vi "太阳能控制器界面.vi"() -> ()   [LabVIEW 2016, in "环境动力监测库.lvlib"]
uses:
  <vilib>/Utility/miscctls.llb/LVPointTypeDef.ctl
  <vilib>/Utility/config.llb/NI_LVConfig.lvlib
  <vilib>/ptbypt/NI_PtbyPt.lvlib
panel:
  out "串口":string
  in  "串口启用 2":bool caption="串口启用"
  in  "串口启用":bool
  in  "报警设置":bool
  in  "MPPT-24 串口":refnum<visa-resource-name> caption="MPPT-24"
  in  "MPPT-12 串口":refnum<visa-resource-name> caption="MPPT-12"
  out "充放电信息 2":T1 caption="充放电信息_KWH" {"总累计充电量" format="%.2f"; "当年累计充电量" format="%.2f"; "当月累计充电量" format="%.2f"; "当日累计充电量" format="%.2f"; "当年累计用电量" format="%.2f"; "当月累计用电量" format="%.2f"; "当日累计用电量" format="%.2f"}
  out "状态 2":string caption="状态"
  out "状态":string
  out "充放电信息":T1 caption="充放电信息_KWH" {"总累计充电量" format="%.2f"; "当年累计充电量" format="%.2f"; "当月累计充电量" format="%.2f"; "当日累计充电量" format="%.2f"; "当年累计用电量" format="%.2f"; "当月累计用电量" format="%.2f"; "当日累计用电量" format="%.2f"}
  out "通讯状态 3":bool
  out "通讯状态 2":bool
  out "控制器信息 2":cluster{"设备温度℃":dbl} caption="控制器信息"
  out "直流负载信息 2":cluster{"负载电压V":dbl, "负载电流A":dbl, "负载功率W":dbl} caption="直流负载信息"
  out "蓄电池信息 2":T2 caption="蓄电池信息"
  out "阵列信息 2":cluster{"阵列电压V":dbl, "阵列电流A":dbl, "发电功率W":dbl} caption="阵列信息"
  out "控制器信息":cluster{"设备温度℃":dbl}
  out "直流负载信息":cluster{"负载电压V":dbl, "负载电流A":dbl, "负载功率W":dbl}
  out "蓄电池信息":T2
  out "阵列信息":cluster{"阵列电压V":dbl, "阵列电流A":dbl, "发电功率W":dbl}
  # "MPPT-12"
  # "MPPT-24"
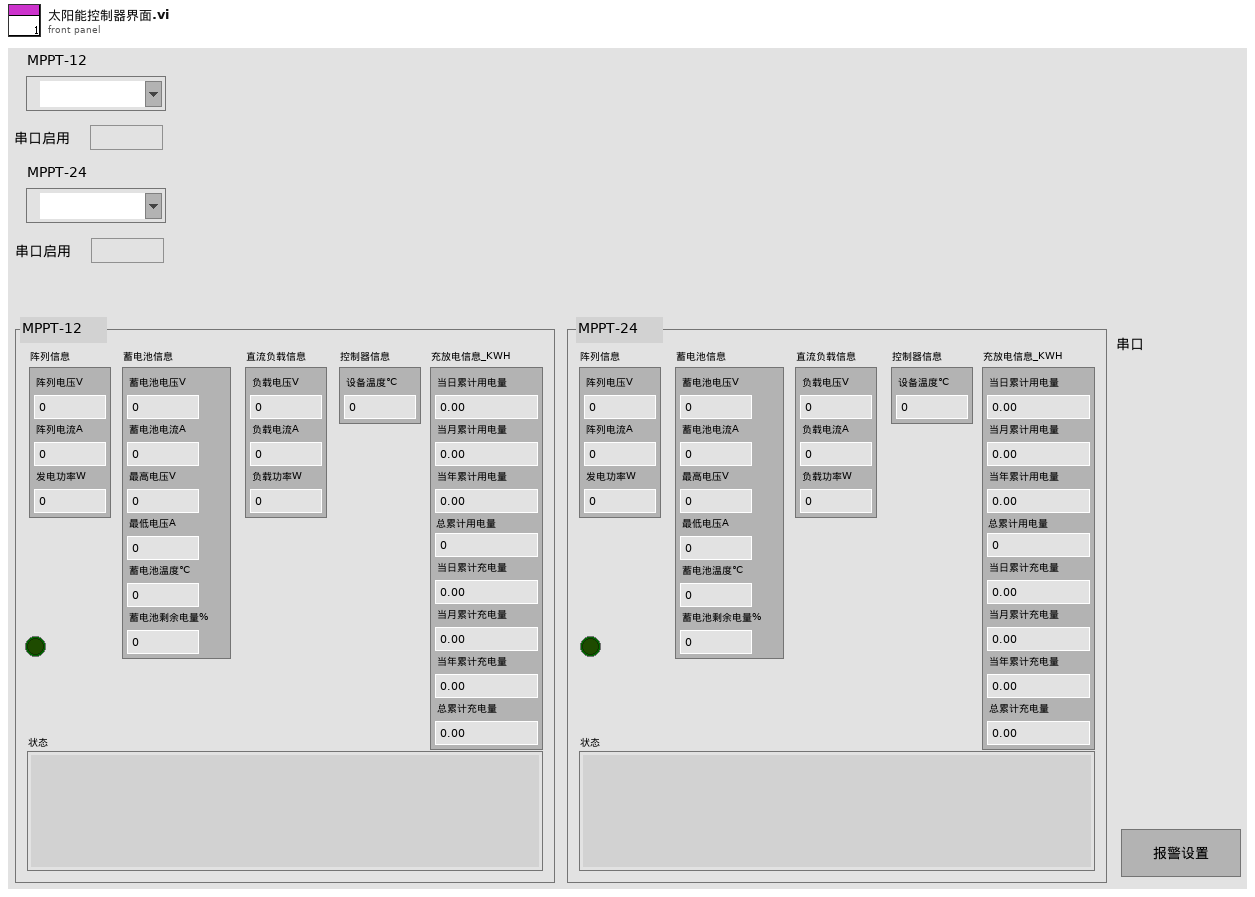
[diagram p1: front panel]
types:
  T1 = cluster{"当日累计用电量":sgl, "当月累计用电量":sgl, "当年累计用电量":sgl, "总累计用电量":sgl, "当日累计充电量":sgl, "当月累计充电量":sgl, "当年累计充电量":sgl, "总累计充电量":sgl}
  T2 = cluster{"蓄电池电压V":dbl, "蓄电池电流A":dbl, "最高电压V":dbl, "最低电压A":dbl, "蓄电池温度℃":dbl, "蓄电池剩余电量%":dbl}
  T3 = cluster{"监测项描述:输出":string, "连接方式":enum16{"串口", "TCP"}, "端口":string, "IP address:":string, "Port:":string, "站号":u64, "传感器型号":string, "波特率":u64, "data bits":u64, "停止位":u16, "奇偶校验":u16}
  T4 = typedef "LVPointTypeDef.ctl" = cluster{"Horizontal":i16, "Vertical":i16}
  T5 = typedef "NI_LVConfig.lvlib/Config Data RefNum.ctl" = refnum<k1>
  T6 = cluster{"时间":timestamp, "阵列电压_V":dbl, "阵列电流_A":dbl, "发电功率_W":dbl, "蓄电池电压_V":dbl, "蓄电池电流_A":dbl, "最高电压_V":dbl, "最低电压_A":dbl, "蓄电池温度_℃":dbl, "蓄电池剩余电量_%":dbl, "负载电压_V":dbl, "负载电流_A":dbl, "负载功率_W":dbl, "设备温度_℃":dbl, "当日累计用电量_KWH":dbl, "当月累计用电量_KWH":dbl, "当年累计用电量_KWH":dbl, "总累计用电量_KWH":dbl, "当日累计充电量_KWH":dbl, "当月累计充电量_KWH":dbl, "当年累计充电量_KWH":dbl, "总累计充电量_KWH":dbl}
  T7 = typedef "LVDateTimeRec.ctl" = cluster{"秒数的小数部分":dbl, "秒":i32, "分":i32, "时":i32, "日":i32, "月":i32, "年":i32, "天数（周）":i32, "天数（年）":i32, "DST":i32}
  T8 = cluster{"漏水监测输出":bool, "门禁监测输出":bool, "温湿度监测输出":bool, "烟雾监测输出":bool, "空调监测输出":bool, "自动重合闸输出":bool, "红外入侵输出":bool, "振动输出":bool, "UPS输出":bool, "蓄电池输出":bool, "定位输出":bool}
  T9 = cluster{"状态":cluster{"蓄电池状态":string, "阵列状态":string, "充电状态":string, "负载状态":string, "设备状态":string}, "充放电信息":cluster{"当日累计用电量":sgl, "当月累计用电量":sgl, "当年累计用电量":sgl, "总累计用电量":sgl, "当日累计充电量":sgl, "当月累计充电量":sgl, "当年累计充电量":sgl, "总累计充电量":sgl}, "控制器信息":cluster{"设备温度℃":dbl}, "蓄电池信息":cluster{"蓄电池电压V":dbl, "蓄电池电流A":dbl, "最高电压V":dbl, "最低电压A":dbl, "蓄电池温度℃":dbl, "蓄电池剩余电量%":dbl}, "阵列信息":cluster{"阵列电压V":dbl, "阵列电流A":dbl, "发电功率W":dbl}, "直流负载信息":cluster{"负载电压V":dbl, "负载电流A":dbl, "负载功率W":dbl}, "error out":errorcluster}
  T10 = cluster{"市电":cluster{"电压:":u16, "电流：":dbl, "状态":bool}, "UPS":cluster{"输入电压:":sgl, "输出电压:":sgl, "电池电量:":u8, "电量":u16, "状态":bool}, "蓄电池":cluster{"电压:":sgl, "电流:":sgl, "电池电量:":u8, "电量":u16, "状态":bool}}
  T11 = enum8{"Enabled", "Disabled", "Disabled and Grayed Out"}
  T12 = cluster{"蓄电池状态":string, "阵列状态":string, "充电状态":string, "负载状态":string, "设备状态":string}
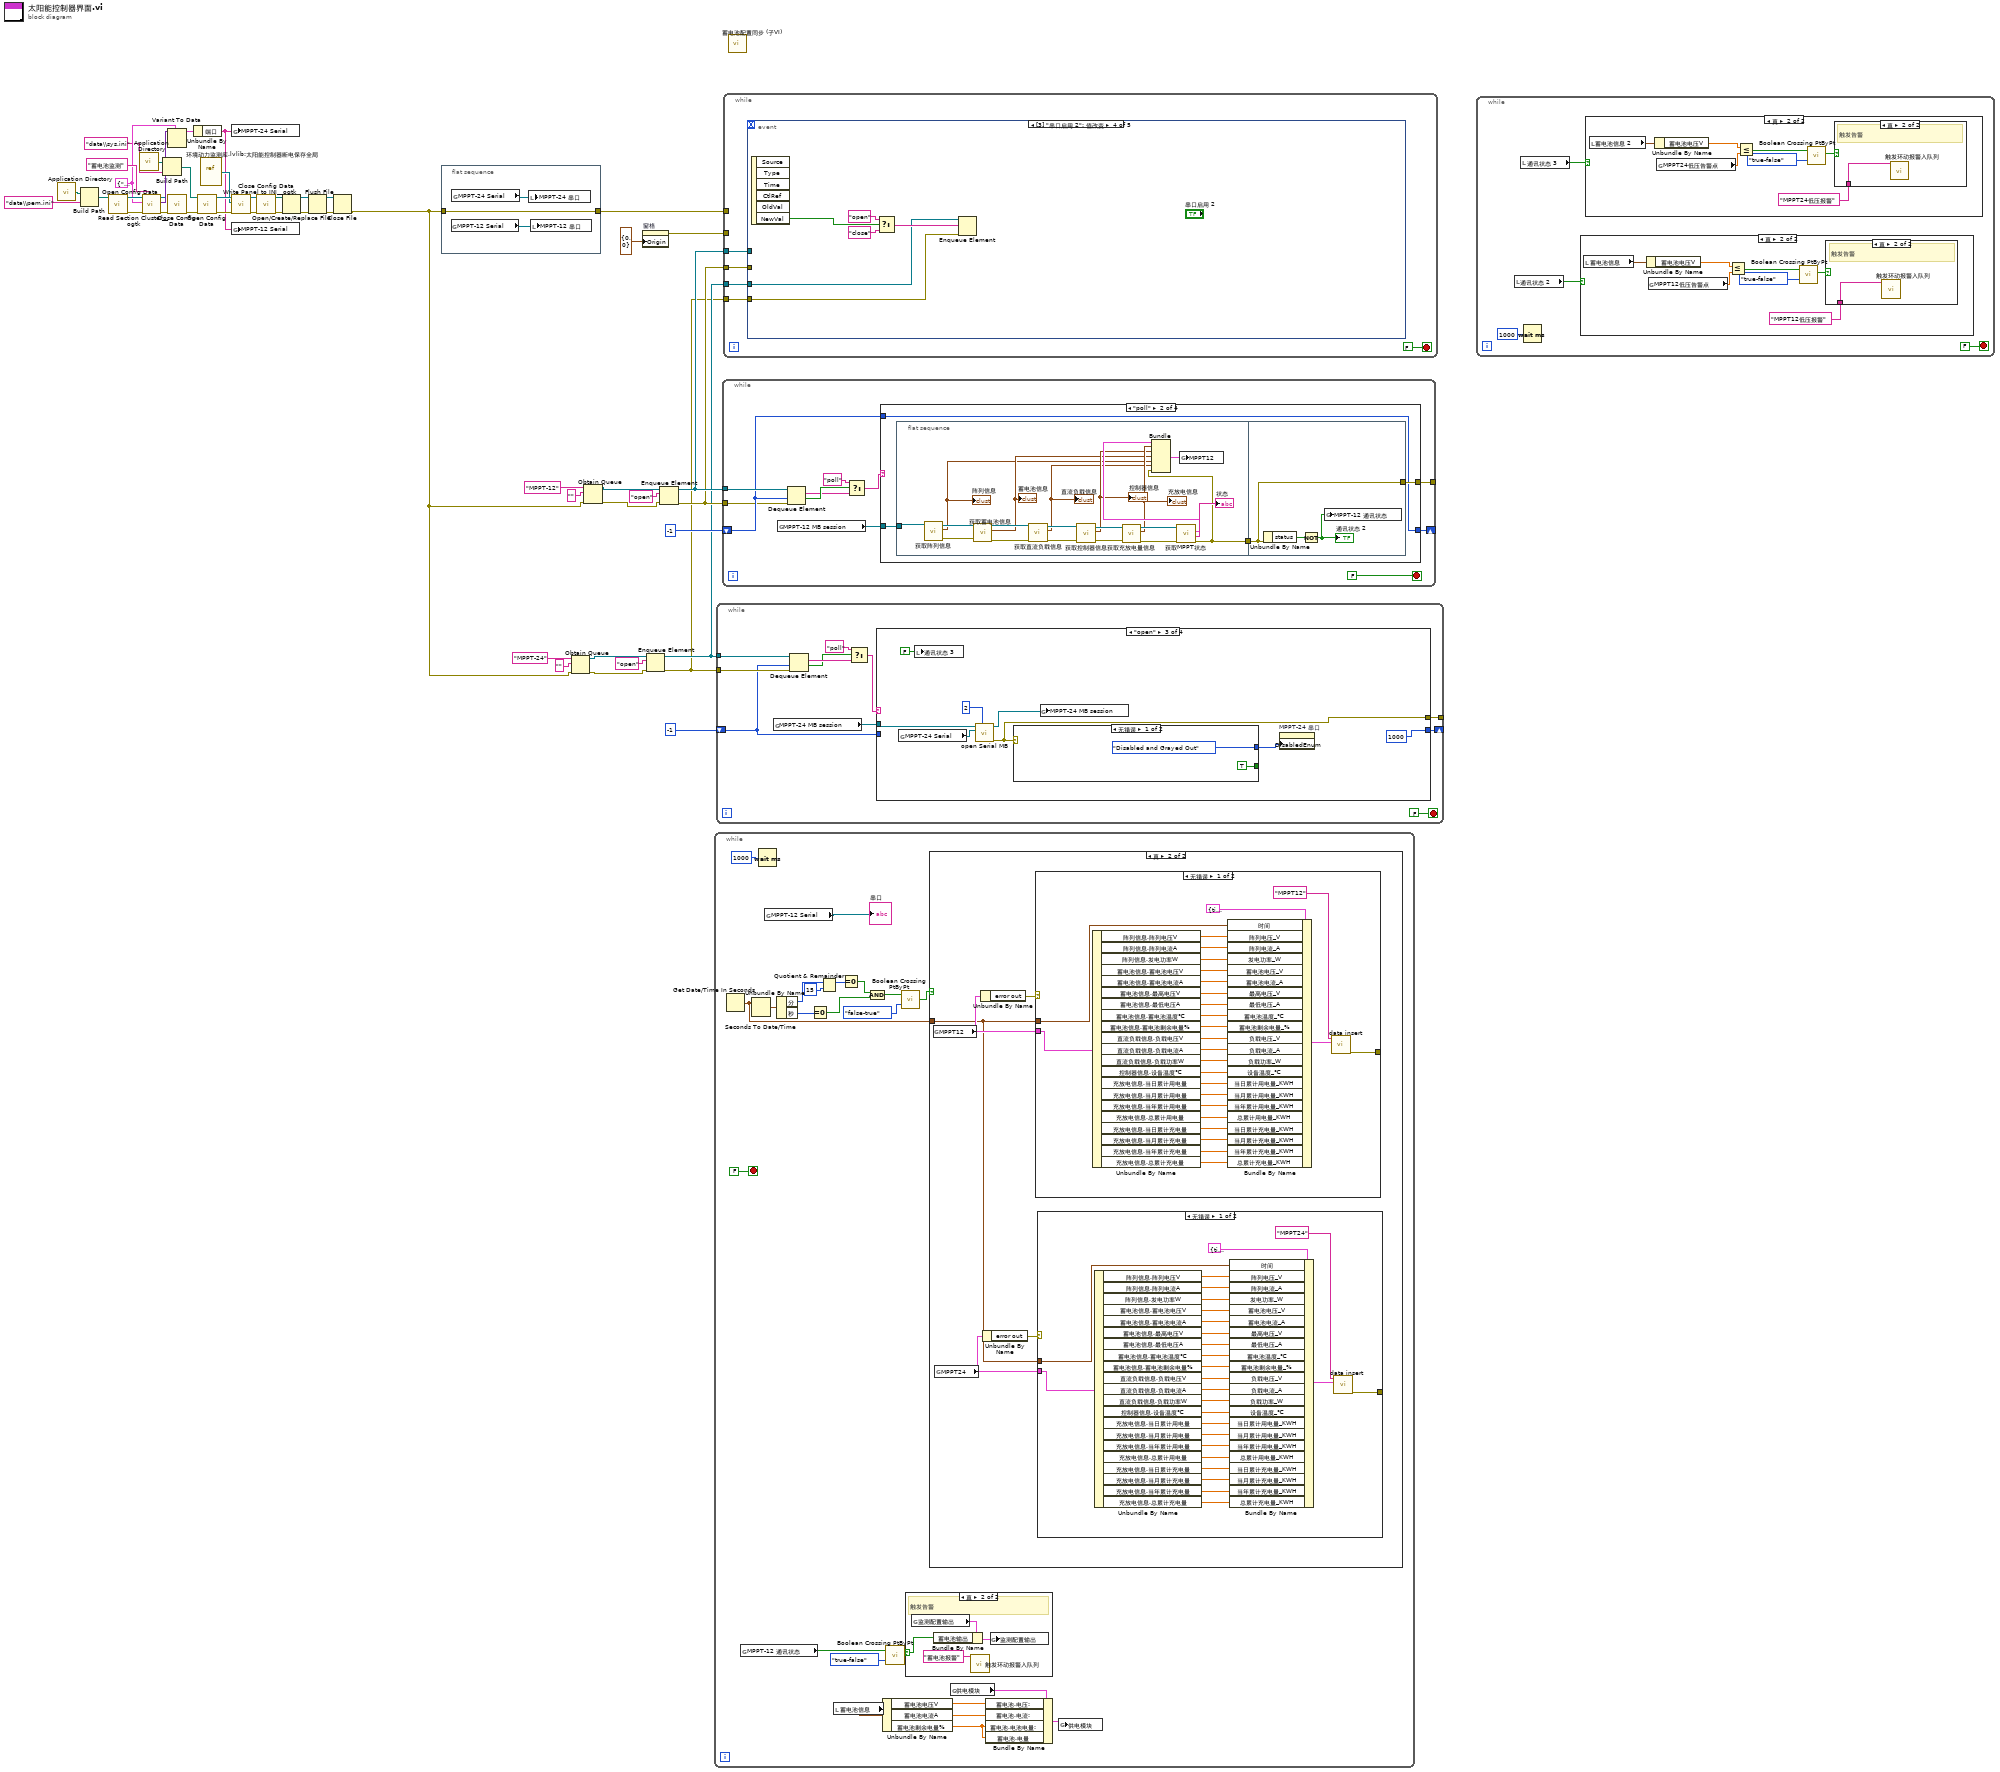
[diagram p0: block diagram]
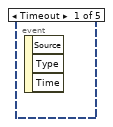
[diagram p10: hidden frame]
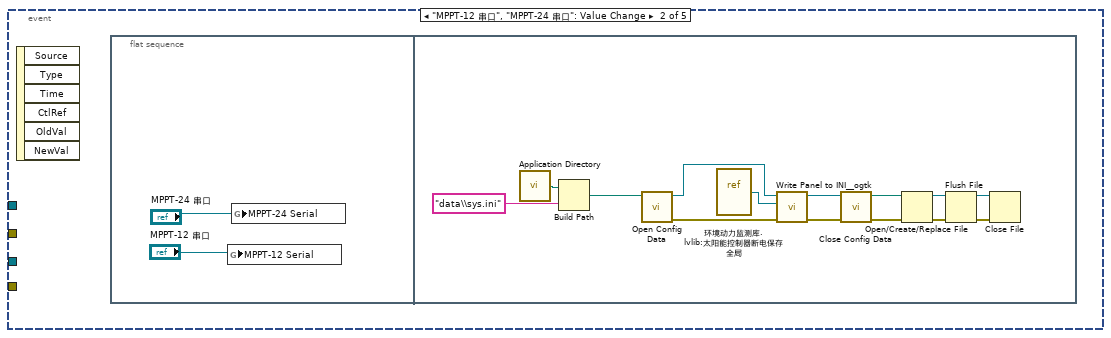
[diagram p11: hidden frame]
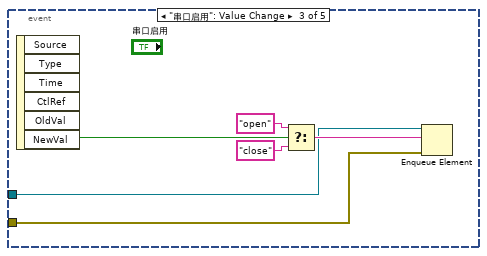
[diagram p12: hidden frame]
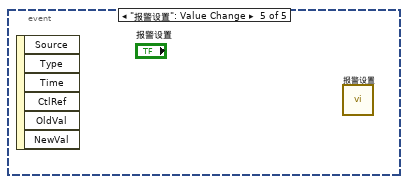
[diagram p13: hidden frame]
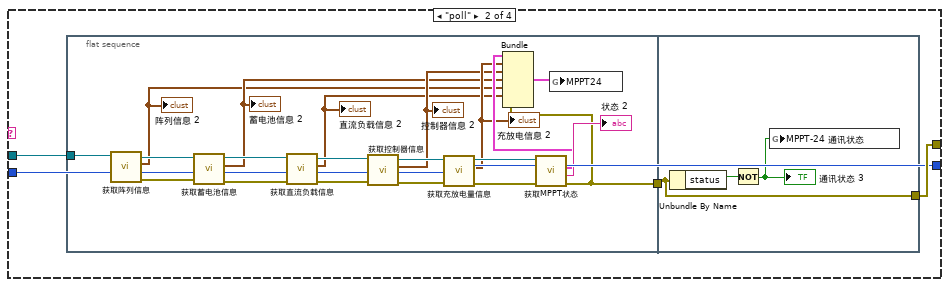
[diagram p15: hidden frame]
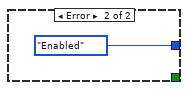
[diagram p16: hidden frame]
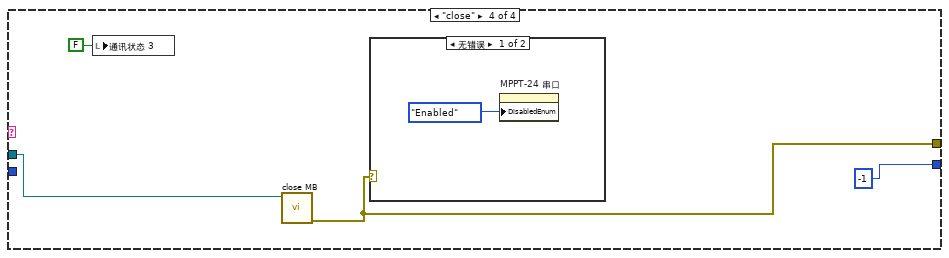
[diagram p17: hidden frame]
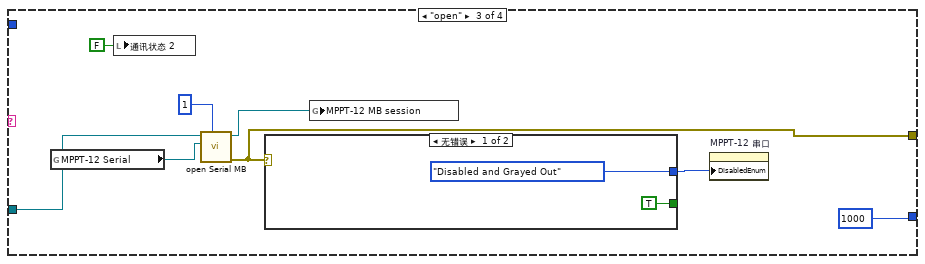
[diagram p20: hidden frame]
diagram:
  w18 = T3 {"监测项描述:输出"="", "连接方式"=enum."串口", "端口"="", "IP address:"="", "Port:"="", "站号"=19200, "传感器型号"="", "波特率"=19200, "data bits"=8, "停止位"=10, "奇偶校验"=0} ("输入簇")
  n1 = call <vilib>:"Application Directory.vi"() -> ("Application Directory"=w22:path)
  n2 = Build Path(base path=w22, name or relative path="data\\pem.ini" ("名称或相对路径")) -> (appended path=w21:path)
  n3 = call <vilib>:"Open Config Data.vi"("configuration file path"=w21) -> ("error out"=w20:errorcluster, "refnum"=w19:T5)  [unwired: 8 in, 1 out]
  n4 = call <vilib>:"Application Directory.vi"() -> ("Application Directory"=w16:path)
  n5 = call <userlib>:"Read Section Cluster__ogtk.vi"("section (optional)"="蓄电池监测", "error in (no error)"=w20, "Section Formatted Cluster Type"=w18, "refnum"=w19) -> ("error out"=w26:errorcluster, "Section Formatted Cluster"=w27:variant, "dup refnum"=w25:T5)  [unwired: 3 in, 2 out]
  n6 = Build Path(base path=w16, name or relative path="data\\sys.ini" ("名称或相对路径")) -> (appended path=w15:path)
  n7 = Variant To Data(type=w18, Variant=w27) -> (data=w28:T3)  [unwired: 1 in, 1 out]
  n8 = call <vilib>:"Close Config Data.vi"("error in (no error)"=w26, "refnum"=w25) -> ("error out"=w4:errorcluster)  [unwired: 8 in, 1 out]
  n9 = Unbundle By Name(w28) -> ("端口"=w2:string)
  n10 = call <vilib>:"Open Config Data.vi"("error in (no error)"=w4, "configuration file path"=w15) -> ("error out"=w12:errorcluster, "refnum"=w14:T5)  [unwired: 7 in, 1 out]
  n11 = vi-ref "环境动力监测库.lvlib:太阳能控制器断电保存全局.vi"() -> (w3:refnum<vi>)
  n12 = global write "太阳能控制器断电保存全局.vi" "MPPT-24 Serial"(w2) -> ()
  n13 = call <userlib>:"Write Panel to INI__ogtk.vi"("error in (no error)"=w12, "VI ref"=w3, "refnum"=w14) -> ("error out"=w11:errorcluster, "refnum out"=w13:T5)  [unwired: 7 in]
  n14 = global write "太阳能控制器断电保存全局.vi" "MPPT-12 Serial"(w2) -> ()
  n15 = call <vilib>:"Close Config Data.vi"("error in (no error)"=w11, "refnum"=w13) -> ("error out"=w6:errorcluster, "file path"=w5:path)  [unwired: 8 in]
  n16 = Open/Create/Replace File(file path (use dialog)=w5, error in=w6) -> (refnum out=w9:refnum<file>, error out=w10:errorcluster)  [unwired: 4 in, 1 out]
  n17 = Flush File(refnum=w9, error in=w10) -> (refnum out=w8:refnum<file>, error out=w7:errorcluster)
  n18 = Close File(refnum=w8, error in=w7) -> (error out=w1:errorcluster)  [unwired: 1 out]
  n19 = flat-sequence {
    tunnel: w1 -> [w48]
    tunnel: [w48] -> w33
    frame #0 {
      n20 = global read "太阳能控制器断电保存全局.vi" "MPPT-12 Serial"() -> (w50:refnum<visa-resource-name>)
      n21 = global read "太阳能控制器断电保存全局.vi" "MPPT-24 Serial"() -> (w49:refnum<visa-resource-name>)
      n22 = local write "MPPT-24 串口"(w49) -> ()
      n23 = local write "MPPT-12 串口"(w50) -> ()
    }
  }
  n24 = Obtain Queue(name (unnamed)="MPPT-24" ("名称（未命名）"), element data type="", error in (no error)=w1) -> (queue out=w35:refnum<queue>, error out=w34:errorcluster)  [unwired: 2 in, 1 out]
  n25 = Obtain Queue(name (unnamed)="MPPT-12" ("名称（未命名）"), element data type="", error in (no error)=w1) -> (queue out=w37:refnum<queue>, error out=w36:errorcluster)  [unwired: 2 in, 1 out]
  n26 = property on="窗格" class="Pane"("Origin"=T4 {"Horizontal"=0, "Vertical"=0} ("原点")) -> (error out=w44:errorcluster)  [unwired: 2 in, 1 out]
  n27 = Enqueue Element(queue=w35, element="open" ("元素"), error in (no error)=w34) -> (queue out=w30:refnum<queue>, error out=w29:errorcluster)  [unwired: 1 in, 1 out]
  n28 = Enqueue Element(queue=w37, element="open" ("元素"), error in (no error)=w36) -> (queue out=w32:refnum<queue>, error out=w31:errorcluster)  [unwired: 1 in, 1 out]
  n29 = while {
    stop <- FALSE stop-if-true
    n30 = Get Date/Time In Seconds() -> (seconds since 1Jan1904=w61:timestamp)
    n31 = global read "太阳能控制器全局.vi" "MPPT-12 通讯状态"() -> (w51:bool)
    n32 = Seconds To Date/Time(time stamp (now)=w61) -> (date time rec=w71:T7)  [unwired: 1 in]
    n33 = Wait (ms)(milliseconds to wait=u32 1000 ("等待时间（毫秒）")) -> ()  [unwired: 1 out]
    n34 = global read "太阳能控制器断电保存全局.vi" "MPPT-12 Serial"() -> (→"串口":refnum<visa-resource-name>)
    n35 = Unbundle By Name(w71) -> ("分"=w70:i32, "秒"=w67:i32)
    n36 = Equal To 0?(x=w67) -> (x = 0?=w65:bool)
    n37 = Quotient & Remainder(x=w70, y=15) -> (x-y*floor(x/y)=w68:i32)  [unwired: 1 out]
    n38 = local read "蓄电池信息"() -> (w55:T2)
    n39 = Equal To 0?(x=w68) -> (x = 0?=w66:bool)
    n40 = And(x=w66, y=w65) -> (x .and. y?=w64:bool)
    n41 = Unbundle By Name(w55) -> ("蓄电池电压V"=w54:dbl, "蓄电池电流A"=w53:dbl, "蓄电池剩余电量%"=w52:dbl)
    n42 = call <vilib>:"Boolean Crossing PtByPt.vi"("direction"=enum16{"either", "false-true", "true-false"}."true-false", "input"=w51) -> ("crossing"=w58:bool)  [unwired: 1 in]
    n43 = call <vilib>:"Boolean Crossing PtByPt.vi"("direction"=enum16{"either", "false-true", "true-false"}."false-true", "input"=w64) -> ("crossing"=w62:bool)  [unwired: 1 in]
    n44 = case shown="真" w58 {
      selector: w58 -> [_ w74]
      frame False {
      }
      frame True {
        # "触发告警"
        n45 = global read "断电保存全局变量.vi" "监测配置输出"() -> (w76:T8)
        n46 = Bundle By Name(cluster=w76, "蓄电池输出"=w74) -> (w75:T8)
        n47 = call "触发环动报警入队列.vi"("报警内容"="蓄电池报警") -> ()  [unwired: 11 in]
        n48 = global write "断电保存全局变量.vi" "监测配置输出"(w75) -> ()
      }
    }
    n49 = case shown="真" w62 {
      tunnel: w61 -> [_ w78]
      frame False {
      }
      frame True {
        n50 = global read "太阳能控制器全局.vi" "MPPT12"() -> (w81:T9)
        n51 = global read "太阳能控制器全局.vi" "MPPT24"() -> (w80:T9)
        n52 = Unbundle By Name(w81) -> ("error out"=w82:errorcluster)
        n53 = Unbundle By Name(w80) -> ("error out"=w79:errorcluster)
        n54 = case shown="无错误" w82 {
          tunnel: w81 -> [w114 _]
          tunnel: w78 -> [w113 _]
          tunnel: [w110 _] -> _
          frame No Error {
            n55 = Unbundle By Name(w114) -> ("阵列信息.阵列电压V"=w116:dbl, "阵列信息.阵列电流A"=w117:dbl, "阵列信息.发电功率W"=w118:dbl, "蓄电池信息.蓄电池电压V"=w119:dbl, "蓄电池信息.蓄电池电流A"=w120:dbl, "蓄电池信息.最高电压V"=w121:dbl, "蓄电池信息.最低电压A"=w122:dbl, "蓄电池信息.蓄电池温度℃"=w123:dbl, "蓄电池信息.蓄电池剩余电量%"=w124:dbl, "直流负载信息.负载电压V"=w125:dbl, "直流负载信息.负载电流A"=w126:dbl, "直流负载信息.负载功率W"=w127:dbl, "控制器信息.设备温度℃"=w128:dbl, "充放电信息.当日累计用电量"=w129:sgl, "充放电信息.当月累计用电量"=w130:sgl, "充放电信息.当年累计用电量"=w131:sgl, "充放电信息.总累计用电量"=w132:sgl, "充放电信息.当日累计充电量"=w133:sgl, "充放电信息.当月累计充电量"=w134:sgl, "充放电信息.当年累计充电量"=w135:sgl, "充放电信息.总累计充电量"=w136:sgl)
            n56 = Bundle By Name(cluster=T6 {"时间"=timestamp(0 s since 1904-01-01), "阵列电压_V"=0.0, "阵列电流_A"=0.0, "发电功率_W"=0.0, "蓄电池电压_V"=0.0, "蓄电池电流_A"=0.0, "最高电压_V"=0.0, "最低电压_A"=0.0, "蓄电池温度_℃"=0.0, "蓄电池剩余电量_%"=0.0, "负载电压_V"=0.0, "负载电流_A"=0.0, "负载功率_W"=0.0, "设备温度_℃"=0.0, "当日累计用电量_KWH"=0.0, "当月累计用电量_KWH"=0.0, "当年累计用电量_KWH"=0.0, "总累计用电量_KWH"=0.0, "当日累计充电量_KWH"=0.0, "当月累计充电量_KWH"=0.0, "当年累计充电量_KWH"=0.0, "总累计充电量_KWH"=0.0} ("data in"), "时间"=w113, "阵列电压_V"=w116, "阵列电流_A"=w117, "发电功率_W"=w118, "蓄电池电压_V"=w119, "蓄电池电流_A"=w120, "最高电压_V"=w121, "最低电压_A"=w122, "蓄电池温度_℃"=w123, "蓄电池剩余电量_%"=w124, "负载电压_V"=w125, "负载电流_A"=w126, "负载功率_W"=w127, "设备温度_℃"=w128, "当日累计用电量_KWH"=w129, "当月累计用电量_KWH"=w130, "当年累计用电量_KWH"=w131, "总累计用电量_KWH"=w132, "当日累计充电量_KWH"=w133, "当月累计充电量_KWH"=w134, "当年累计充电量_KWH"=w135, "总累计充电量_KWH"=w136) -> (w112:T6)
            n57 = call "data insert.vi"("data in"=w112, "table"="MPPT12") -> ("error out"=w110:errorcluster)  [unwired: 9 in]
          }
          frame Error {
          }
        }
        n58 = case shown="无错误" w79 {
          tunnel: w80 -> [w87 _]
          tunnel: w78 -> [w86 _]
          tunnel: [w83 _] -> _
          frame No Error {
            n59 = Unbundle By Name(w87) -> ("阵列信息.阵列电压V"=w89:dbl, "阵列信息.阵列电流A"=w90:dbl, "阵列信息.发电功率W"=w91:dbl, "蓄电池信息.蓄电池电压V"=w92:dbl, "蓄电池信息.蓄电池电流A"=w93:dbl, "蓄电池信息.最高电压V"=w94:dbl, "蓄电池信息.最低电压A"=w95:dbl, "蓄电池信息.蓄电池温度℃"=w96:dbl, "蓄电池信息.蓄电池剩余电量%"=w97:dbl, "直流负载信息.负载电压V"=w98:dbl, "直流负载信息.负载电流A"=w99:dbl, "直流负载信息.负载功率W"=w100:dbl, "控制器信息.设备温度℃"=w101:dbl, "充放电信息.当日累计用电量"=w102:sgl, "充放电信息.当月累计用电量"=w103:sgl, "充放电信息.当年累计用电量"=w104:sgl, "充放电信息.总累计用电量"=w105:sgl, "充放电信息.当日累计充电量"=w106:sgl, "充放电信息.当月累计充电量"=w107:sgl, "充放电信息.当年累计充电量"=w108:sgl, "充放电信息.总累计充电量"=w109:sgl)
            n60 = Bundle By Name(cluster=T6 {"时间"=timestamp(0 s since 1904-01-01), "阵列电压_V"=0.0, "阵列电流_A"=0.0, "发电功率_W"=0.0, "蓄电池电压_V"=0.0, "蓄电池电流_A"=0.0, "最高电压_V"=0.0, "最低电压_A"=0.0, "蓄电池温度_℃"=0.0, "蓄电池剩余电量_%"=0.0, "负载电压_V"=0.0, "负载电流_A"=0.0, "负载功率_W"=0.0, "设备温度_℃"=0.0, "当日累计用电量_KWH"=0.0, "当月累计用电量_KWH"=0.0, "当年累计用电量_KWH"=0.0, "总累计用电量_KWH"=0.0, "当日累计充电量_KWH"=0.0, "当月累计充电量_KWH"=0.0, "当年累计充电量_KWH"=0.0, "总累计充电量_KWH"=0.0} ("data in"), "时间"=w86, "阵列电压_V"=w89, "阵列电流_A"=w90, "发电功率_W"=w91, "蓄电池电压_V"=w92, "蓄电池电流_A"=w93, "最高电压_V"=w94, "最低电压_A"=w95, "蓄电池温度_℃"=w96, "蓄电池剩余电量_%"=w97, "负载电压_V"=w98, "负载电流_A"=w99, "负载功率_W"=w100, "设备温度_℃"=w101, "当日累计用电量_KWH"=w102, "当月累计用电量_KWH"=w103, "当年累计用电量_KWH"=w104, "总累计用电量_KWH"=w105, "当日累计充电量_KWH"=w106, "当月累计充电量_KWH"=w107, "当年累计充电量_KWH"=w108, "总累计充电量_KWH"=w109) -> (w85:T6)
            n61 = call "data insert.vi"("data in"=w85, "table"="MPPT24") -> ("error out"=w83:errorcluster)  [unwired: 9 in]
          }
          frame Error {
          }
        }
      }
    }
    n62 = global read "内部交互全局变量.vi" "供电模块"() -> (w57:T10)
    n63 = Bundle By Name(cluster=w57, "蓄电池.电压:"=w54, "蓄电池.电流:"=w53, "蓄电池.电池电量:"=w52, "蓄电池.电量"=w52) -> (w56:T10)
    n64 = global write "内部交互全局变量.vi" "供电模块"(w56) -> ()
  }
  n65 = while {
    tunnel: w30 -> [w144]
    tunnel: w29 -> [w143]
    shift-right: [w139] -> _
    shift-left: -1 ("超时毫秒(-1)") -> [w137]
    tunnel: [w140] -> _
    stop <- FALSE stop-if-true
    n66 = global read "太阳能控制器全局.vi" "MPPT-24 MB session"() -> (w141:refnum<class "MB_Master.lvclass">)
    n67 = Dequeue Element(queue=w144, timeout in ms (-1)=w137, error in (no error)=w143) -> (element=w147:string, timed out?=w145:bool)  [unwired: 2 out]
    n68 = Select(t="poll" ("元素"), s=w145, f=w147) -> (s? t:f=w142:string)
    n69 = case shown="\"open\"" w142 {
      tunnel: w141 -> [_ w152 w179 w189]
      tunnel: [_ w150 w178 w188] -> w140
      tunnel: [w148 w149 1000 ("超时毫秒(-1)") -1 ("超时毫秒(-1)")] -> w139
      tunnel: w137 -> [w148 w149 _ _]
      frame Default {
      }
      frame "poll" {
        n70 = flat-sequence {
          tunnel: w152 -> [w162]
          tunnel: [w153] -> w151
          tunnel: w151 -> [w173]
          tunnel: [w173] -> w150
          frame #0 {
            n71 = call "获取阵列信息.vi"("MB session in"=w162) -> ("error out"=w171:errorcluster, "阵列信息"=w155:cluster{"阵列电压V":dbl, "阵列电流A":dbl, "发电功率W":dbl}, "MB session out"=w172:refnum<class "MB_Master.lvclass">)  [unwired: 8 in]
            "阵列信息 2" <- w155
            n72 = call "获取蓄电池信息.vi"("error in (no error)"=w171, "MB session in"=w172) -> ("error out"=w169:errorcluster, "蓄电池信息"=w156:T2, "MB session out"=w170:refnum<class "MB_Master.lvclass">)  [unwired: 7 in]
            "蓄电池信息 2" <- w156
            n73 = call "获取直流负载信息.vi"("error in (no error)"=w169, "MB session in"=w170) -> ("error out"=w167:errorcluster, "直流负载信息"=w154:cluster{"负载电压V":dbl, "负载电流A":dbl, "负载功率W":dbl}, "MB session out"=w168:refnum<class "MB_Master.lvclass">)  [unwired: 7 in]
            "直流负载信息 2" <- w154
            n74 = call "获取控制器信息.vi"("error in (no error)"=w167, "MB session in"=w168) -> ("error out"=w165:errorcluster, "控制器信息"=w157:cluster{"设备温度℃":dbl}, "MB session out"=w166:refnum<class "MB_Master.lvclass">)  [unwired: 7 in]
            "控制器信息 2" <- w157
            n75 = call "获取充放电量信息.vi"("error in (no error)"=w165, "MB session in"=w166) -> ("error out"=w163:errorcluster, "充放电信息"=w158:T1, "MB session out"=w164:refnum<class "MB_Master.lvclass">)  [unwired: 7 in]
            "充放电信息 2" <- w158
            n76 = call "获取MPPT状态.vi"("error in (no error)"=w163, "MB session in"=w164) -> ("error out"=w153:errorcluster, "结果字符串"=→"状态 2":string, "状态"=w160:T12)  [unwired: 6 in, 1 out]
            n77 = Bundle("状态"=w160, "充放电信息"=w158, "控制器信息"=w157, "蓄电池信息"=w156, "阵列信息"=w155, "直流负载信息"=w154, "error out"=w153) -> (w159:T9)  [unwired: 1 in]
            n78 = global write "太阳能控制器全局.vi" "MPPT24"(w159) -> ()
          }
          frame #1 {
            n79 = Unbundle By Name(w173) -> ("status"=w175:bool)
            n80 = Not(x=w175) -> (.not. x?=w174:bool)
            "通讯状态 3" <- w174
            n81 = global write "太阳能控制器全局.vi" "MPPT-24 通讯状态"(w174) -> ()
          }
        }
      }
      frame "open" {
        n82 = global read "太阳能控制器断电保存全局.vi" "MPPT-24 Serial"() -> (w181:refnum<visa-resource-name>)
        n83 = local write "通讯状态 3"(FALSE ("通讯状态 3")) -> ()
        n84 = call "open Serial MB.vi"("Slave ID"=u8 2, "VISA Resource"=w181, "MB session in"=w179) -> ("error out"=w178:errorcluster, "MB session out"=w182:refnum<class "MB_Master.lvclass">)  [unwired: 7 in]
        n85 = case shown="无错误" w178 {
          tunnel: [T11."Disabled and Grayed Out" ("禁用") T11."Enabled" ("禁用")] -> w176
          tunnel: [TRUE _] -> _
          frame No Error {
          }
          frame Error {
          }
        }
        n86 = global write "太阳能控制器全局.vi" "MPPT-24 MB session"(w182) -> ()
        n87 = property on="MPPT-24 串口" class="VISAName"("DisabledEnum"=w176) -> ()  [unwired: 2 in, 2 out]
      }
      frame "close" {
        n88 = local write "通讯状态 3"(FALSE ("通讯状态 2")) -> ()
        n89 = call "close MB.vi"("MB session in"=w189) -> ("error out"=w188:errorcluster)  [unwired: 10 in]
        n90 = case shown="无错误" w188 {
          frame No Error {
            n91 = property on="MPPT-24 串口" class="VISAName"("DisabledEnum"=T11."Enabled" ("禁用")) -> ()  [unwired: 2 in, 2 out]
          }
          frame Error {
          }
        }
      }
    }
  }
  n92 = while {
    shift-right: [w193] -> _
    shift-left: -1 ("超时毫秒(-1)") -> [w194]
    tunnel: w32 -> [w199]
    tunnel: [w195] -> _
    tunnel: w31 -> [w192]
    stop <- FALSE stop-if-true
    n93 = global read "太阳能控制器全局.vi" "MPPT-12 MB session"() -> (w196:refnum<class "MB_Master.lvclass">)
    n94 = Dequeue Element(queue=w199, timeout in ms (-1)=w194, error in (no error)=w192) -> (element=w200:string, timed out?=w202:bool)  [unwired: 2 out]
    n95 = Select(t="poll" ("元素"), s=w202, f=w200) -> (s? t:f=w197:string)
    n96 = case shown="\"poll\"" w197 {
      tunnel: w196 -> [_ w207 w237 w244]
      tunnel: [_ w205 w233 w242] -> w195
      tunnel: w194 -> [w203 w204 _ _]
      tunnel: [w203 w204 1000 ("超时毫秒(-1)") -1 ("超时毫秒(-1)")] -> w193
      frame Default {
      }
      frame "poll" {
        n97 = flat-sequence {
          tunnel: w207 -> [w227]
          tunnel: [w209] -> w206
          tunnel: w206 -> [w228]
          tunnel: [w228] -> w205
          frame #0 {
            n98 = call "获取阵列信息.vi"("MB session in"=w227) -> ("error out"=w225:errorcluster, "阵列信息"=w211:cluster{"阵列电压V":dbl, "阵列电流A":dbl, "发电功率W":dbl}, "MB session out"=w226:refnum<class "MB_Master.lvclass">)  [unwired: 8 in]
            "阵列信息" <- w211
            n99 = call "获取蓄电池信息.vi"("error in (no error)"=w225, "MB session in"=w226) -> ("error out"=w223:errorcluster, "蓄电池信息"=w212:T2, "MB session out"=w224:refnum<class "MB_Master.lvclass">)  [unwired: 7 in]
            "蓄电池信息" <- w212
            n100 = call "获取直流负载信息.vi"("error in (no error)"=w223, "MB session in"=w224) -> ("error out"=w221:errorcluster, "直流负载信息"=w210:cluster{"负载电压V":dbl, "负载电流A":dbl, "负载功率W":dbl}, "MB session out"=w222:refnum<class "MB_Master.lvclass">)  [unwired: 7 in]
            "直流负载信息" <- w210
            n101 = call "获取控制器信息.vi"("error in (no error)"=w221, "MB session in"=w222) -> ("error out"=w219:errorcluster, "控制器信息"=w213:cluster{"设备温度℃":dbl}, "MB session out"=w220:refnum<class "MB_Master.lvclass">)  [unwired: 7 in]
            "控制器信息" <- w213
            n102 = call "获取充放电量信息.vi"("error in (no error)"=w219, "MB session in"=w220) -> ("error out"=w217:errorcluster, "充放电信息"=w214:T1, "MB session out"=w218:refnum<class "MB_Master.lvclass">)  [unwired: 7 in]
            "充放电信息" <- w214
            n103 = call "获取MPPT状态.vi"("error in (no error)"=w217, "MB session in"=w218) -> ("error out"=w209:errorcluster, "结果字符串"=→"状态":string, "状态"=w215:T12)  [unwired: 6 in, 1 out]
            n104 = Bundle("状态"=w215, "充放电信息"=w214, "控制器信息"=w213, "蓄电池信息"=w212, "阵列信息"=w211, "直流负载信息"=w210, "error out"=w209) -> (w208:T9)  [unwired: 1 in]
            n105 = global write "太阳能控制器全局.vi" "MPPT12"(w208) -> ()
          }
          frame #1 {
            n106 = Unbundle By Name(w228) -> ("status"=w230:bool)
            n107 = Not(x=w230) -> (.not. x?=w229:bool)
            "通讯状态 2" <- w229
            n108 = global write "太阳能控制器全局.vi" "MPPT-12 通讯状态"(w229) -> ()
          }
        }
      }
      frame "open" {
        n109 = global read "太阳能控制器断电保存全局.vi" "MPPT-12 Serial"() -> (w231:refnum<visa-resource-name>)
        n110 = local write "通讯状态 2"(FALSE ("通讯状态 2")) -> ()
        n111 = call "open Serial MB.vi"("Slave ID"=u8 1, "VISA Resource"=w231, "MB session in"=w237) -> ("error out"=w233:errorcluster, "MB session out"=w235:refnum<class "MB_Master.lvclass">)  [unwired: 7 in]
        n112 = case shown="无错误" w233 {
          tunnel: [T11."Disabled and Grayed Out" ("禁用") T11."Enabled" ("禁用")] -> w234
          tunnel: [TRUE _] -> _
          frame No Error {
          }
          frame Error {
          }
        }
        n113 = global write "太阳能控制器全局.vi" "MPPT-12 MB session"(w235) -> ()
        n114 = property on="MPPT-12 串口" class="VISAName"("DisabledEnum"=w234) -> ()  [unwired: 2 in, 2 out]
      }
      frame "close" {
        n115 = local write "通讯状态 2"(FALSE ("通讯状态 2")) -> ()
        n116 = call "close MB.vi"("MB session in"=w244) -> ("error out"=w242:errorcluster)  [unwired: 10 in]
        n117 = case shown="无错误" w242 {
          frame No Error {
            n118 = property on="MPPT-12 串口" class="VISAName"("DisabledEnum"=T11."Enabled" ("禁用")) -> ()  [unwired: 2 in, 2 out]
          }
          frame Error {
          }
        }
      }
    }
  }
  n119 = while {
    tunnel: w44 -> [_]
    tunnel: w33 -> [_]
    tunnel: w32 -> [w250]
    tunnel: w31 -> [w249]
    tunnel: w30 -> [w248]
    tunnel: w29 -> [w247]
    stop <- FALSE stop-if-true
    n120 = event shown="[3] \"串口启用 2\": 值改变" {
      selector: _ -> [_ _ _ _ _]
      dyn-events: _ -> [_ _ _ _ _]
      timeout: _ -> [_ _ _ _ _]
      tunnel: w250 -> [_ _ w269 _ _]
      tunnel: w249 -> [_ _ w268 _ _]
      tunnel: w248 -> [_ _ _ w275 _]
      tunnel: w247 -> [_ _ _ w274 _]
      event Timeout {
        n121 = event-data() -> ()  [unwired: 1 in, 3 out]
      }
      event "MPPT-12 串口", "MPPT-24 串口": Value Change {
        n122 = event-data() -> ()  [unwired: 1 in, 6 out]
        n123 = flat-sequence {
          frame #0 {
            n124 = global write "太阳能控制器断电保存全局.vi" "MPPT-12 Serial"("MPPT-12 串口") -> ()
            n125 = global write "太阳能控制器断电保存全局.vi" "MPPT-24 Serial"("MPPT-24 串口") -> ()
          }
          frame #1 {
            n126 = call <vilib>:"Application Directory.vi"() -> ("Application Directory"=w267:path)
            n127 = Build Path(base path=w267, name or relative path="data\\sys.ini" ("名称或相对路径")) -> (appended path=w265:path)
            n128 = call <vilib>:"Open Config Data.vi"("configuration file path"=w265) -> ("error out"=w261:errorcluster, "refnum"=w264:T5)  [unwired: 8 in, 1 out]
            n129 = vi-ref "环境动力监测库.lvlib:太阳能控制器断电保存全局.vi"() -> (w263:refnum<vi>)
            n130 = call <userlib>:"Write Panel to INI__ogtk.vi"("error in (no error)"=w261, "VI ref"=w263, "refnum"=w264) -> ("error out"=w260:errorcluster, "refnum out"=w262:T5)  [unwired: 7 in]
            n131 = call <vilib>:"Close Config Data.vi"("error in (no error)"=w260, "refnum"=w262) -> ("error out"=w255:errorcluster, "file path"=w254:path)  [unwired: 8 in]
            n132 = Open/Create/Replace File(file path (use dialog)=w254, error in=w255) -> (refnum out=w258:refnum<file>, error out=w259:errorcluster)  [unwired: 4 in, 1 out]
            n133 = Flush File(refnum=w258, error in=w259) -> (refnum out=w257:refnum<file>, error out=w256:errorcluster)
            n134 = Close File(refnum=w257, error in=w256) -> ()  [unwired: 2 out]
          }
        }
      }
      event "串口启用": Value Change {
        n135 = event-data() -> ("NewVal"=w270:bool)  [unwired: 1 in, 5 out]
        n136 = Select(t="open", s=w270, f="close") -> (s? t:f=w272:string)
        n137 = Enqueue Element(queue=w269, element=w272, error in (no error)=w268) -> ()  [unwired: 1 in, 3 out]
      }
      event "串口启用 2": Value Change {
        n138 = event-data() -> ("NewVal"=w276:bool)  [unwired: 1 in, 5 out]
        n139 = Select(t="open", s=w276, f="close") -> (s? t:f=w278:string)
        n140 = Enqueue Element(queue=w275, element=w278, error in (no error)=w274) -> ()  [unwired: 1 in, 3 out]
      }
      event "报警设置": Value Change {
        n141 = event-data() -> ()  [unwired: 1 in, 6 out]
        n142 = call "报警设置.vi"() -> ()  [unwired: 12 in]
      }
    }
  }
  n143 = call "蓄电池配置同步 (子VI).vi"() -> ()  [unwired: 12 in]
  n144 = while {
    stop <- FALSE stop-if-true
    n145 = local read "通讯状态 2"() -> (w281:bool)
    n146 = local read "通讯状态 3"() -> (w280:bool)
    n147 = Wait (ms)(milliseconds to wait=u32 1000 ("等待时间（毫秒）")) -> ()  [unwired: 1 out]
    n148 = case shown="真" w281 {
      frame False {
      }
      frame True {
        n149 = local read "蓄电池信息"() -> (w298:T2)
        n150 = Unbundle By Name(w298) -> ("蓄电池电压V"=w295:dbl)
        n151 = global read "太阳能控制器断电保存全局.vi" "MPPT12低压告警点"() -> (w294:dbl)
        n152 = Less Or Equal?(x=w295, y=w294) -> (x <= y?=w293:bool)
        n153 = call <vilib>:"Boolean Crossing PtByPt.vi"("direction"=enum16{"either", "false-true", "true-false"}."true-false", "input"=w293) -> ("crossing"=w296:bool)  [unwired: 1 in]
        n154 = case shown="真" w296 {
          tunnel: "MPPT12低压报警" ("设备") -> [_ w299]
          frame False {
          }
          frame True {
            # "触发告警"
            n155 = call "触发环动报警入队列.vi"("报警内容"=w299) -> ()  [unwired: 11 in]
          }
        }
      }
    }
    n156 = case shown="真" w280 {
      frame False {
      }
      frame True {
        n157 = local read "蓄电池信息 2"() -> (w290:T2)
        n158 = Unbundle By Name(w290) -> ("蓄电池电压V"=w287:dbl)
        n159 = global read "太阳能控制器断电保存全局.vi" "MPPT24低压告警点"() -> (w286:dbl)
        n160 = Less Or Equal?(x=w287, y=w286) -> (x <= y?=w285:bool)
        n161 = call <vilib>:"Boolean Crossing PtByPt.vi"("direction"=enum16{"either", "false-true", "true-false"}."true-false", "input"=w285) -> ("crossing"=w288:bool)  [unwired: 1 in]
        n162 = case shown="真" w288 {
          tunnel: "MPPT24低压报警" ("设备") -> [_ w291]
          frame False {
          }
          frame True {
            # "触发告警"
            n163 = call "触发环动报警入队列.vi"("报警内容"=w291) -> ()  [unwired: 11 in]
          }
        }
      }
    }
  }
